vi "PWM Servo position RT.vi"() -> ()   [LabVIEW 2014]
doc: "This VI shows an example of how to implement a closed loop position move using the NI 9505. The position loop is implemented using PID. The output of the loop is used as the command for the current loop, which then sets the PWM duty cycle for the motor. This example assumes that an encoder is connected for position and velocity feedback. This example does not implement advanced motion features such as trajectory generation and splining."
uses:
  <vilib>/LabVIEW Targets/FPGA/cRIO/cRIO-9505/controls.llb/_nicrio_cRIO-9505_DriveStatus.ctl
  <vilib>/FPGAPlugInAG/cRIO-9074/niLvFpga_Open_cRIO-9074.vi
  <vilib>/Utility/error.llb/Error Cluster From Error Code.vi
  <vilib>/rvi/errors/niLvFpgaAdjustHostInterfaceError.vi
  <vilib>/FPGAPlugInAG/cRIO-9074/niLvFpga_Close_cRIO-9074.vi
  <vilib>/rvi/interface/nirviOpenFPGA/nirviOpenFPGA.xnode
  FPGA Bitfiles/MotorLabAProject_FPGATarget_PWMServoposition_WfmhZmwB8YY.lvbitx
  <vilib>/rvi/interface/nirviReadWriteControl/nirviReadWriteControl.xnode
  <vilib>/rvi/interface/nirviCloseFPGA/nirviCloseFPGA.xnode
  NiFpgaLv.dll
panel:
  out "Max Encoder Position":i32
  out "Waveform Chart":T1(graph)
  out "error out":errorcluster
  out "Drive Status":T2=enum."Disabled"
  in  "Current PI Gains":T3={"Proportional Gain"=20, "Integral Gain"=10, "Derivative Gain"=0}
  in  "Current Limit (Amps)":dbl=1.0 min=0.0 max=12.0
  in  "Current Loop Rate (usec)":u32=50
  out "Encoder Position":i32
  out "Position Error Status":bool
  out "Position Error Read":i16
  in  "Position Error Limit":i16=32767
  in  "Position PID Gains":T4={"Kp"=100, "Kd"=1000, "Ki"=0, "ILim"=1000, "Kv"=0, "Vff"=0, "Aff"=0, "Td"=2}
  in  "Position Loop  Rate (usec)":u16=250
  in  "Position Setpoint":i32
  in  "stop":bool
  in  "Reset Position":bool
  in  "Reset Position Value":i32
  # "VI Execution\n1. Set Current Limit (Amps) to an appropriate value for the connected load.\n2. The Current PI Gains and Current Loop Rate (usec) should not need to be changed.\n3. The Position PID Gains are set to default values which should work for most systems. It may be necessary to tune these parameters. If there is concern with the default values, set all gains to 0 prior to running the VI.\n4. Connect an encoder to the 9-pin DSUB connector. See \"NI 9505 Operating Instructions and Specifications\" for pinout information.\n5. Run the VI.\n6. Enter a position to move to in Position Setpoint.\n7. Encoder Position returns the actual position.\n8. Position Error Read returns the difference between  Position Setpoint and Encoder Position.\n9. If the difference between Position Setpoint and Encoder Position is greater than the value in Position Error Limit, the Position Error Status LED will turn on and the move will not be executed."
  # "Kp: 3000\nKd: 2000\nKi: 1000\nILim: 1\n\nProp: 20\nInt: 10\nLoop rate: 50\nLimit: 0.7"
  # "Current Loop Parameters"
  # "Position Loop Parameters"
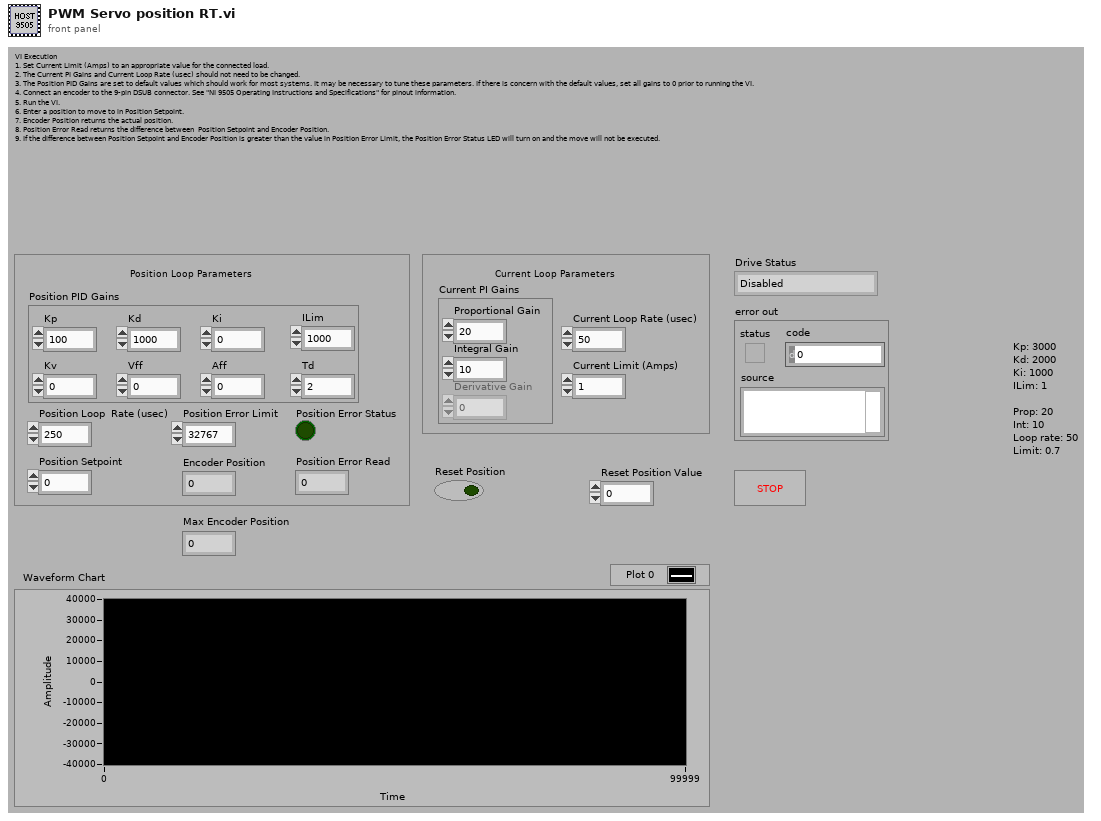
[diagram p1: front panel]
types:
  T1 = cluster{"Position Setpoint":i32, "Encoder Position":i32}
  T2 = typedef "_nicrio_cRIO-9505_DriveStatus.ctl" = enum8{"Enabled", "Disabled", "Disabled by Drive Fault", "Disabled by Temp. Fault", "Disabled by E-Stop", "Unknown"}
  T3 = cluster{"Proportional Gain":i16, "Integral Gain":i16, "Derivative Gain":i16}
  T4 = cluster{"Kp":i16, "Kd":i16, "Ki":i16, "ILim":i16, "Kv":i16, "Vff":i16, "Aff":i16, "Td":i16}
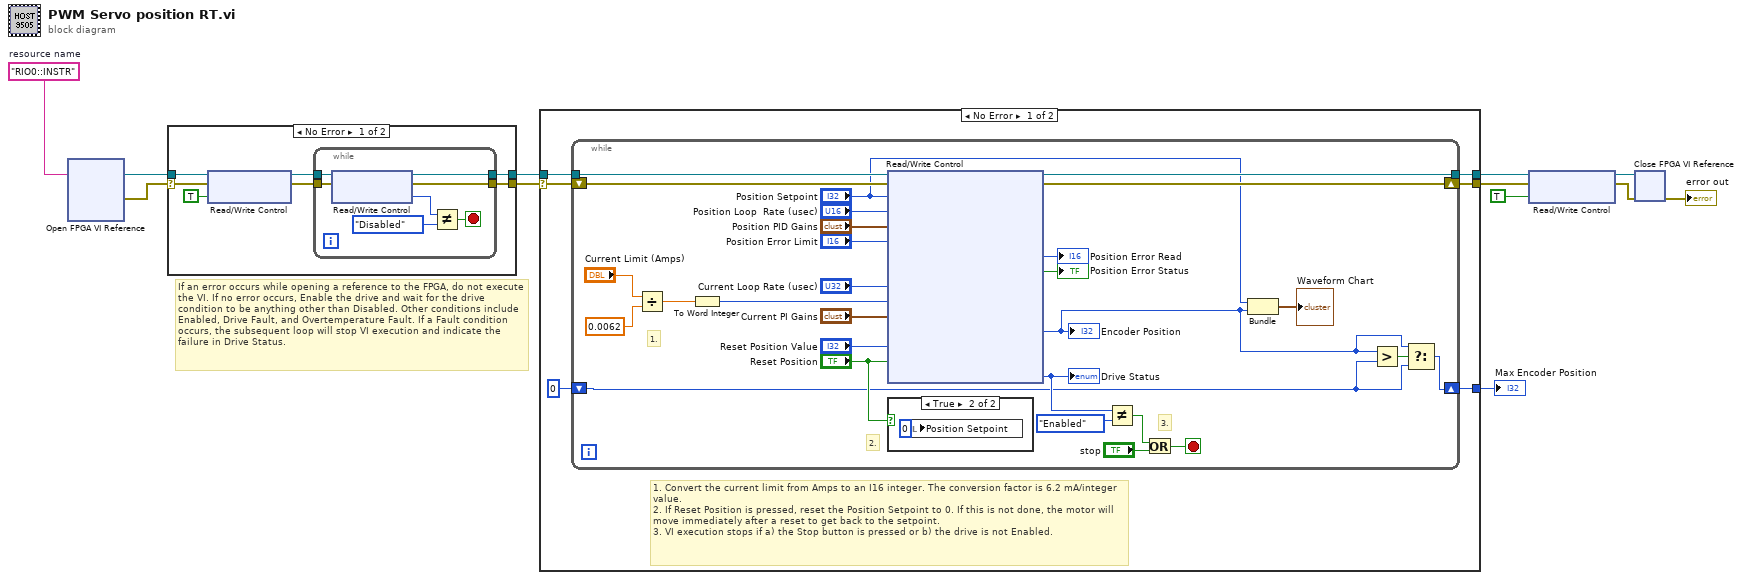
[diagram p0: block diagram]
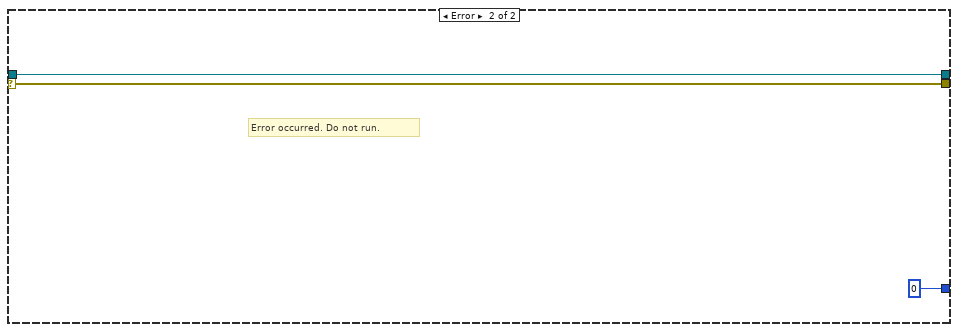
[diagram p4: hidden frame]
diagram:
  w3 = "RIO0::INSTR"  # resource name
  # "If an error occurs while opening a reference to the FPGA, do not execute the VI. If no error occurs, Enable the drive and wait for the drive condition to be anything other than Disabled. Other conditions include Enabled, Drive Fault, and Overtemperature Fault. If a Fault condition occurs, the subsequent loop will stop VI execution and indicate the failure in Drive Status."
  n1 = xnode "Open FPGA VI Reference"("resource name"=w3) -> ("FPGA VI Reference Out"=w6:refnum<k20>, "error out"=w5:errorcluster)  [unwired: 1 in]
  n2 = case shown="No Error" w5 {
    selector: w5 -> [w14 w27]
    tunnel: w6 -> [w17 w28]
    tunnel: [w19 w28] -> w7
    tunnel: [w18 w27] -> w4
    frame No Error {
      n3 = xnode "Read/Write Control"("FPGA VI Reference In"=w17, "error in"=w14, "Enable Drive"=TRUE) -> ("FPGA VI Reference Out"=w16:refnum<k20>, "error out"=w15:errorcluster)
      n4 = while {
        tunnel: [w26] -> w19
        tunnel: [w22] -> w18
        tunnel: w16 -> [w21]
        tunnel: w15 -> [w20]
        stop <- w23 stop-if-true
        n5 = xnode "Read/Write Control"("FPGA VI Reference In"=w21, "error in"=w20) -> ("FPGA VI Reference Out"=w26:refnum<k20>, "error out"=w22:errorcluster, "Drive Status"=w25:T2)
        n6 = Not Equal?(x=w25, y=_nicrio_cRIO-9505_DriveStatus."Disabled") -> (x != y?=w23:bool)
      }
    }
    frame Error {
      # "Error occurred. Do not run."
    }
  }
  n7 = case shown="No Error" w4 {
    selector: w4 -> [w31 w65]
    tunnel: w7 -> [w34 w66]
    tunnel: [w33 w66] -> w12
    tunnel: [w32 w65] -> w11
    tunnel: [w29 0] -> w1
    frame No Error {
      # "1. Convert the current limit from Amps to an I16 integer. The conversion factor is 6.2 mA/integer value.\n2. If Reset Position is pressed, reset the Position Setpoint to 0. If this is not done, the motor will move immediately after a reset to get back to the setpoint.\n3. VI execution stops if a) the Stop button is pressed or b) the drive is not Enabled."
      n8 = while {
        tunnel: w34 -> [w54]
        tunnel: [w52] -> w33
        shift-right: [w51] -> w32
        shift-left: w31 -> [w53]
        shift-right: [w35] -> w29
        shift-left: 0 -> [w38]
        stop <- w50 stop-if-true
        # "3."
        # "1."
        # "2."
        n9 = Divide(x="Current Limit (Amps)", y=0.0062) -> (x/y=w45:dbl)
        n10 = To Word Integer(number=w45) -> (16bit integer=w44:i16)
        n11 = xnode "Read/Write Control"("FPGA VI Reference In"=w54, "error in"=w53, "Position Setpoint"="Position Setpoint", "Position Loop  Rate (usec)"="Position Loop  Rate (usec)", "Position PID Gains"="Position PID Gains", "Position Error Limit"="Position Error Limit", "Current Loop Rate (usec)"="Current Loop Rate (usec)", "Current Limit"=w44, "Current PI Gains"="Current PI Gains", "Reset Position Value"="Reset Position Value", "Reset Position"="Reset Position") -> ("FPGA VI Reference Out"=w52:refnum<k20>, "error out"=w51:errorcluster, "Position Error Read"=→"Position Error Read":i16, "Position Error Status"=→"Position Error Status":bool, "Encoder Position"=w36:i32, "Drive Status"=w43:T2)
        "Encoder Position" <- w36
        "Drive Status" <- w43
        n12 = case shown="True" "Reset Position" {
          frame False {
          }
          frame True {
            n13 = local write "Position Setpoint"(0 ("Position Setpoint")) -> ()
          }
        }
        n14 = Not Equal?(x=w43, y=_nicrio_cRIO-9505_DriveStatus."Enabled") -> (x != y?=w48:bool)
        n15 = Or(x=w48, y="stop") -> (x .or. y?=w50:bool)
        n16 = Bundle("Position Setpoint"="Position Setpoint", "Encoder Position"=w36) -> (→"Waveform Chart":T1)  [unwired: 1 in]
        n17 = Greater?(x=w36, y=w38) -> (0:w37:bool)
        n18 = Select(t=w36, s=w37, f=w38) -> (s? t:f=w35:i32)
      }
    }
    frame Error {
      # "Error occurred. Do not run."
    }
  }
  "Max Encoder Position" <- w1
  n19 = xnode "Read/Write Control"("FPGA VI Reference In"=w12, "error in"=w11, "Disable Drive"=TRUE) -> ("FPGA VI Reference Out"=w10:refnum<k20>, "error out"=w9:errorcluster)
  n20 = xnode "Close FPGA VI Reference"("FPGA VI Reference In"=w10, "error in"=w9) -> ("error out"=→"error out":errorcluster)
